vi "read-device.vi"(8 "error in (no error)":errorcluster, 11 "frameInput in":refnum<class "bFrameIO.lvclass">) -> (0 "error out":errorcluster, 2 "Interface":refnum<k21>, 3 "frameInput out":refnum<class "bFrameIO.lvclass">)   [LabVIEW 2015, in "bFrameIO.lvclass"]
uses:
  bFrameIO.lvclass
  bFrameIO.lvclass/bFrameIO.ctl
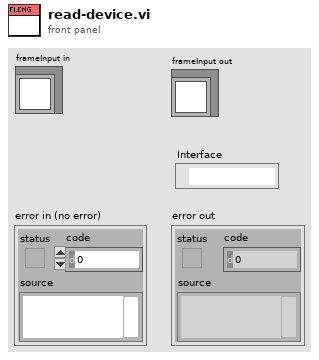
[diagram p1: front panel]
types:
  T1 = typedef "frameInput.lvclass/input.params.ctl" = cluster{"Interface":refnum<k21>, "CAN_Cluster":refnum<k21>, "input.states":T2, "baudrate":u32}
  T2 = typedef "frameInput.lvclass/input-states.ctl" = enum16{"idle", "start", "run", "stop", "exit"}
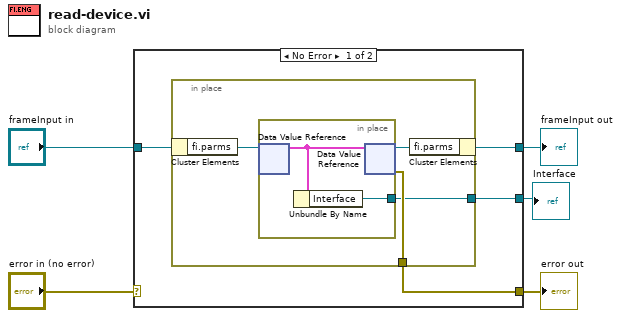
[diagram p0: block diagram]
diagram:
  n1 = case shown="No Error" "error in (no error)" {
    selector: "error in (no error)" -> [_ w16]
    tunnel: [w7 w16] -> w4
    tunnel: [w8 w17] -> w2
    tunnel: "frameInput in" -> [w9 w17]
    tunnel: [w6 _] -> w1
    frame No Error {
      n2 = in-place {
        in-place-border: [w11] -> w7
        in-place-border: [w10] -> w6
        n3 = in-place-cluster #1(w9) -> ("fi.parms"=w13:refnum<data-value>)
        n4 = in-place {
          in-place-border: [w14] -> w10
          n5 = in-place-dvr #2(w13) -> (w15:T1)  [unwired: 1 out]
          n6 = Unbundle By Name(w15) -> ("Interface"=w14:refnum<k21>)
          n7 = in-place-dvr #2(w15) -> (w12:refnum<data-value>, w11:errorcluster)
        }
        n8 = in-place-cluster #1("fi.parms"=w12) -> (w8:refnum<class "bFrameIO.lvclass">)
      }
    }
    frame Error {
    }
  }
  "error out" <- w4
  "frameInput out" <- w2
  "Interface" <- w1
